vi "Main.vi"() -> ()   [LabVIEW 2009]
uses:
  C:/Code/Apps/Utilities/TunableLaserApp/Install/Samples/Labview_TLB-67xx/LabVIEW 2009/UsbDllWrap.dll
panel:
  out "Controller ID":string
  out "Serial Number:":string
  out "Model Number:":string
  out "Calibration Date:":string
  out "bScan":bool
  in  "Lambda Scan":bool
  out "bTrack":bool
  in  "Lambda Track":bool
  out "bLasPwr":bool
  in  "Laser Power":bool
  out "Error Messages":i32(listbox)
  in  "Laser Power Mode":u16(ring) caption="Laser Power" items=["Constant Current", "Constant Power"]
  in  "Stop Wavelength (nm)":dbl format="%.2g"
  in  "Start Wavelength (nm)":dbl format="%.2g"
  in  "Rev. Velocity (nm/s)":dbl format="%.2g"
  in  "Fwd. Velocity (nm/s)":dbl format="%.2g"
  in  "Desired Scans":u16
  out "Scans Completed":dbl
  in  "Piezo Voltage_Set (%)":dbl caption="Piezo Voltage (%)" format="%.2g"
  in  "Power_Set (mW)":dbl caption="Power (mW)" format="%.2g"
  in  "Current_Set (mA)":dbl caption="Current (mA)" format="%.2g"
  in  "Wavelength_Set (nm)":dbl caption="Wavelength (nm)" format="%.2g"
  out "Cavity Temp._Act (degC)":dbl caption="Cavity Temp. (degC)" format="%.2g"
  out "Diode Temp._Act (degC)":dbl caption="Diode Temp. (degC)" format="%.2g"
  out "Power_Act (mW)":dbl caption="Power (mW)" format="%.2g"
  out "Current_Act (mA)":dbl caption="Current (mA)" format="%.2g"
  out "Wavelength_Act (nm)":dbl caption="Wavelength (nm)"
  in  "Selected Controller":u16(ring) items=["6700 P1002", "TLB-6700-XP P1001"]
  # "Actual Values"
  # "Setpoint Values"
  # "Scan Settings"
  # "Mode Settings"
  # "Outputs"
  # "Laser Information"
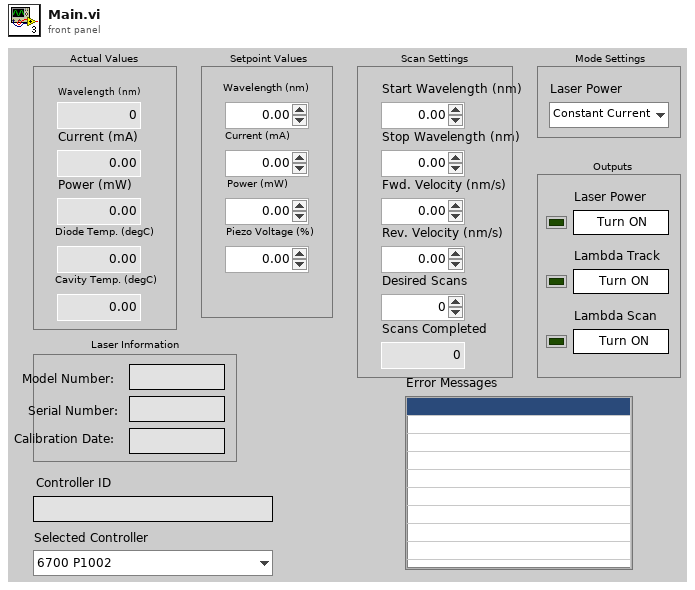
[diagram p1: front panel]
types:
  T1 = cluster{"Laser Power Mode":u16, "Start Wavelength (nm)":dbl, "Stop Wavelength (nm)":dbl, "Fwd. Velocity (nm/s)":dbl, "Rev. Velocity (nm/s)":dbl, "Desired Scans":u16, "Calibration Date:":string, "Model Number:":string, "Serial Number:":string, "Wavelength_Set (nm)":dbl, "Current_Set (mA)":dbl, "Power_Set (mW)":dbl, "Piezo Voltage_Set (%)":dbl, "Controller ID":string}
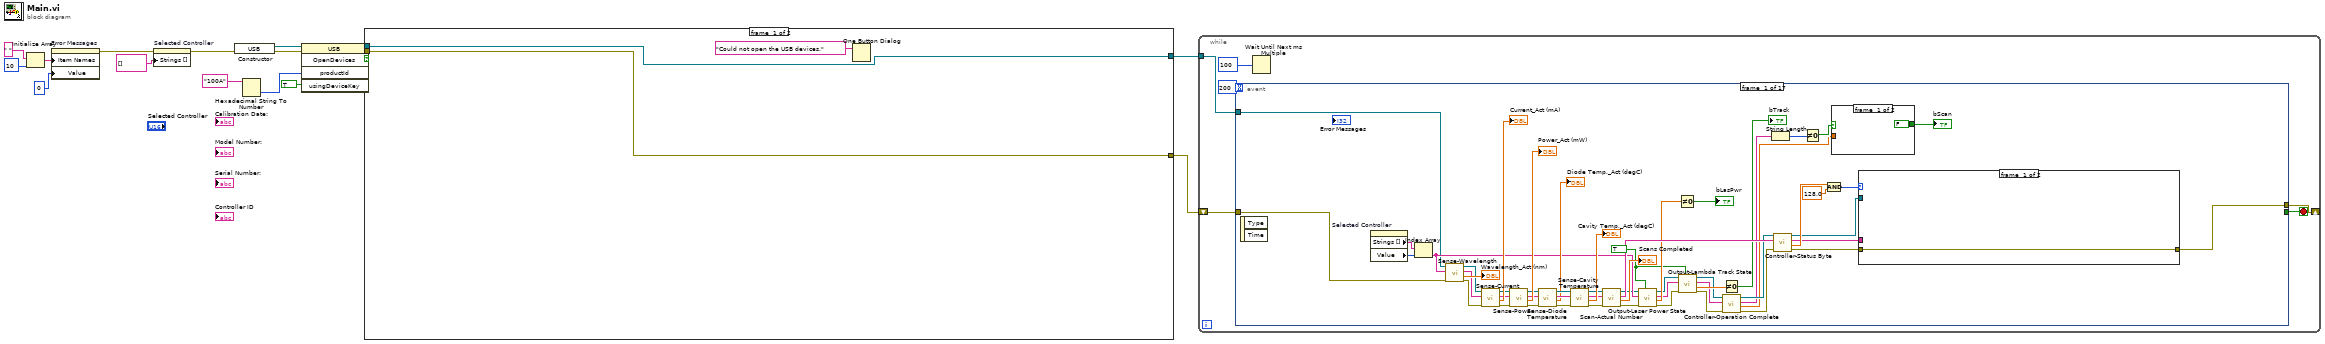
[diagram p0: block diagram]
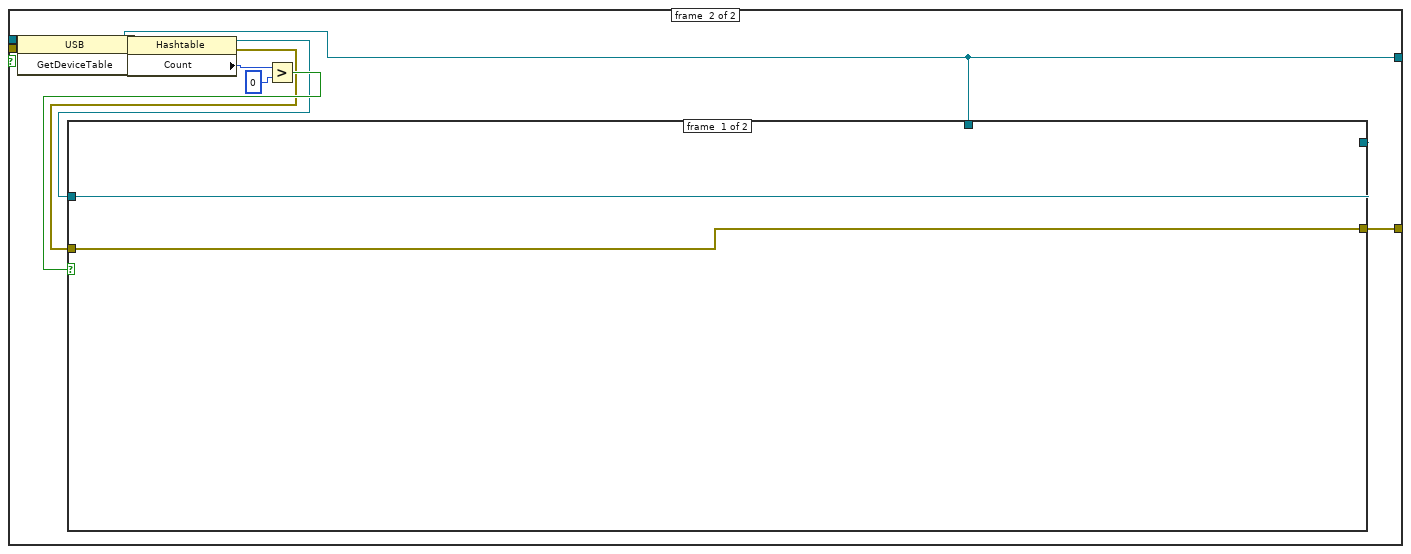
[diagram p2: hidden frame]
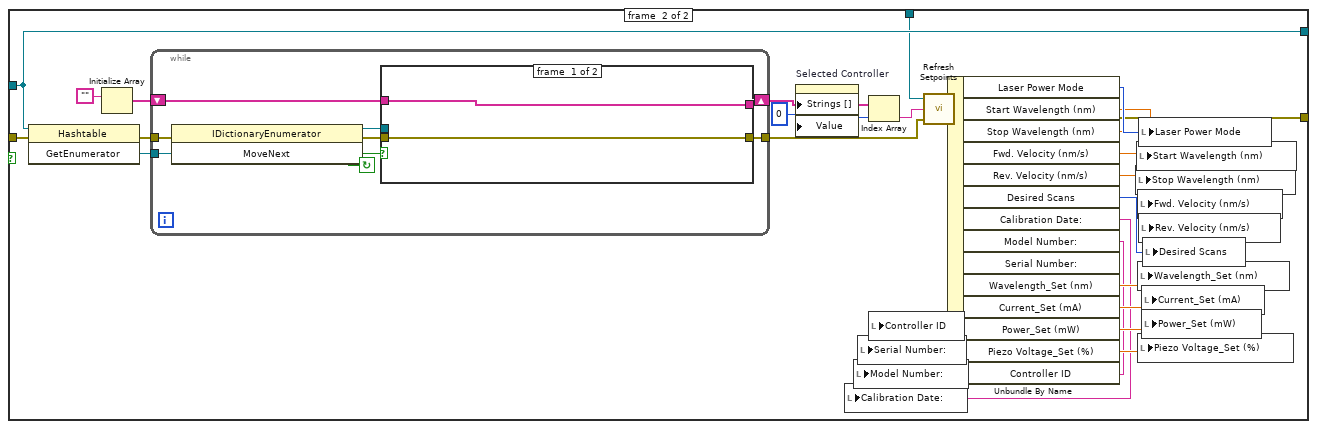
[diagram p3: hidden frame]
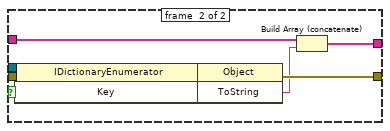
[diagram p4: hidden frame]
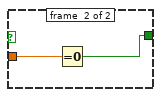
[diagram p5: hidden frame]
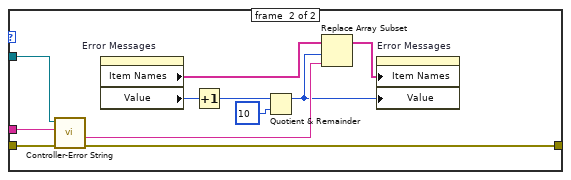
[diagram p6: hidden frame]
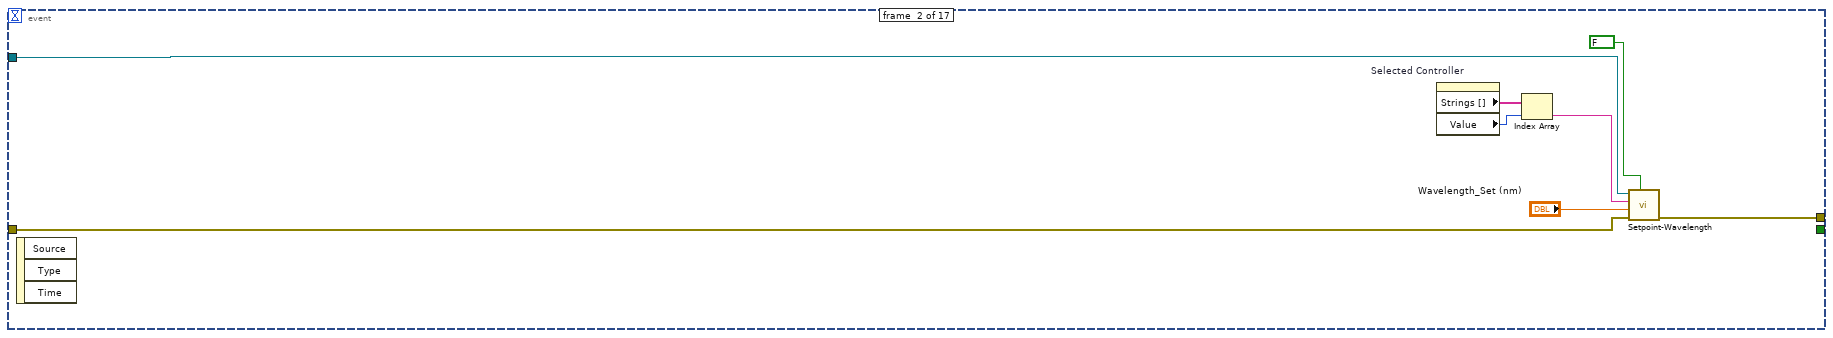
[diagram p7: hidden frame]
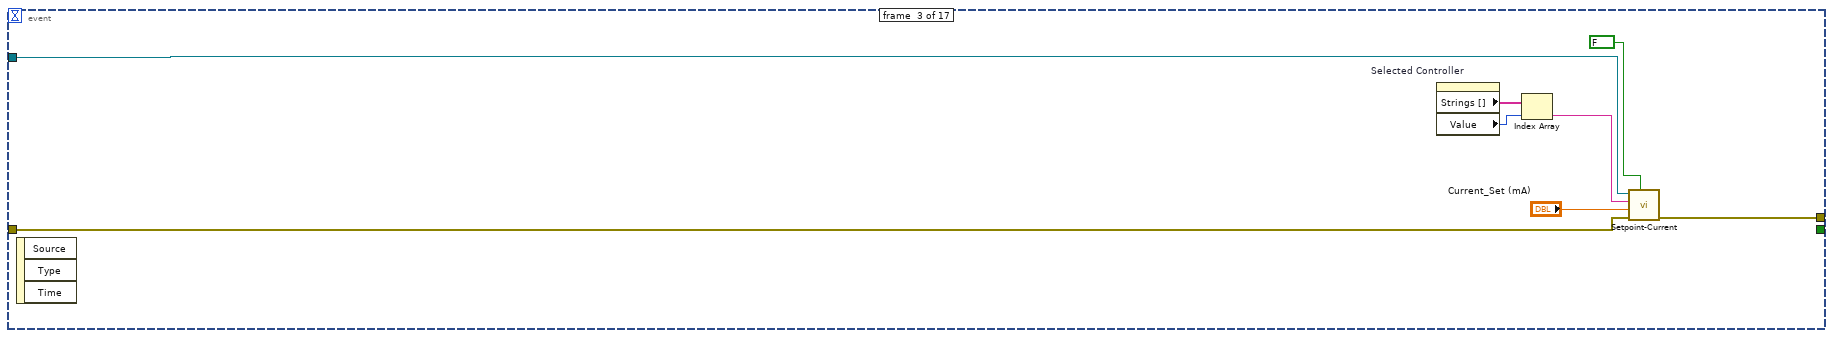
[diagram p8: hidden frame]
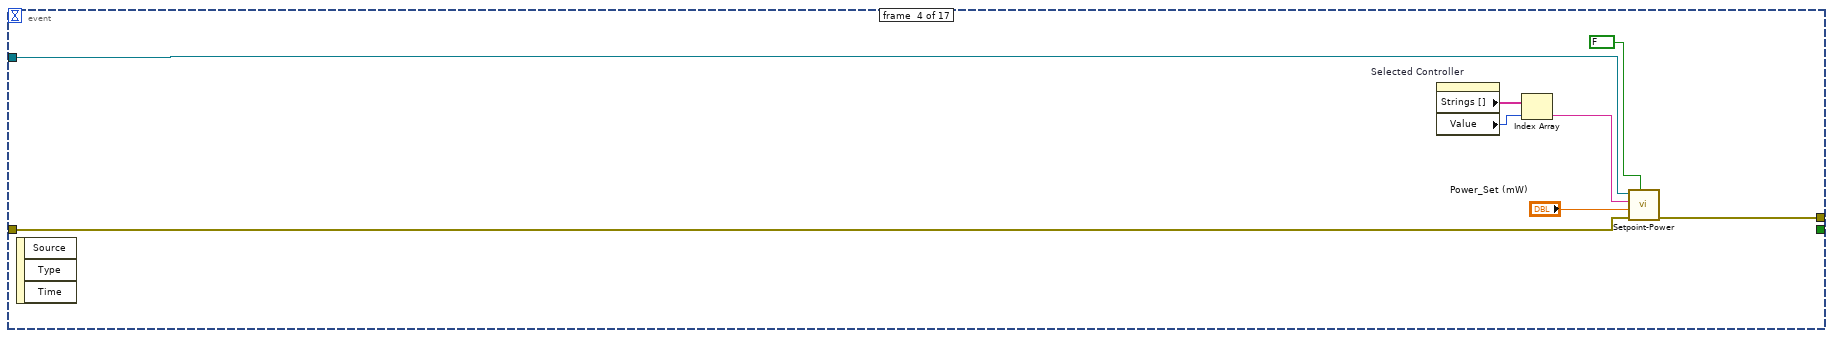
[diagram p9: hidden frame]
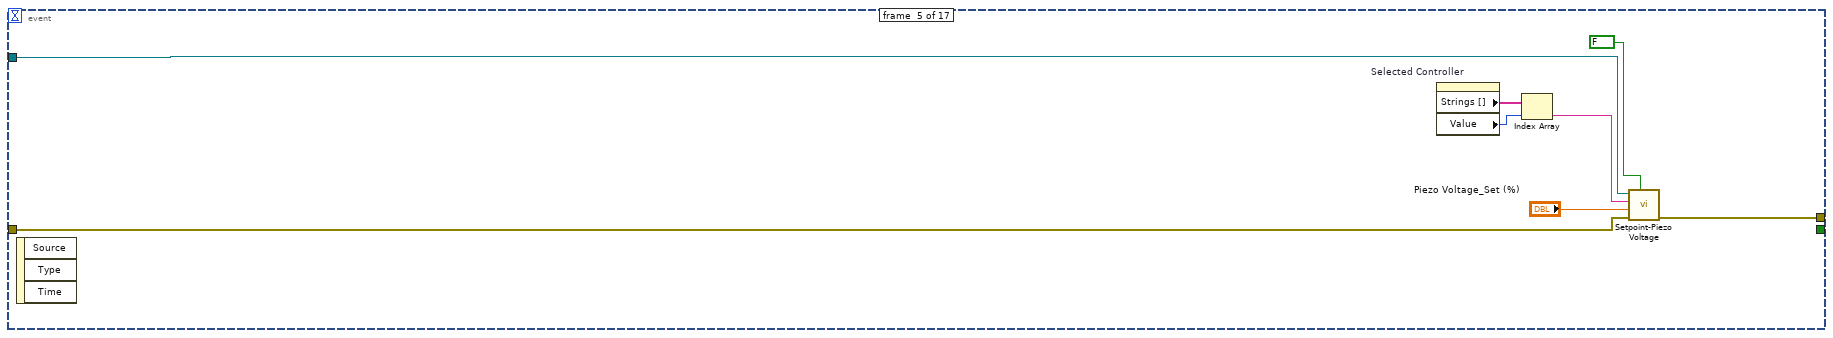
[diagram p10: hidden frame]
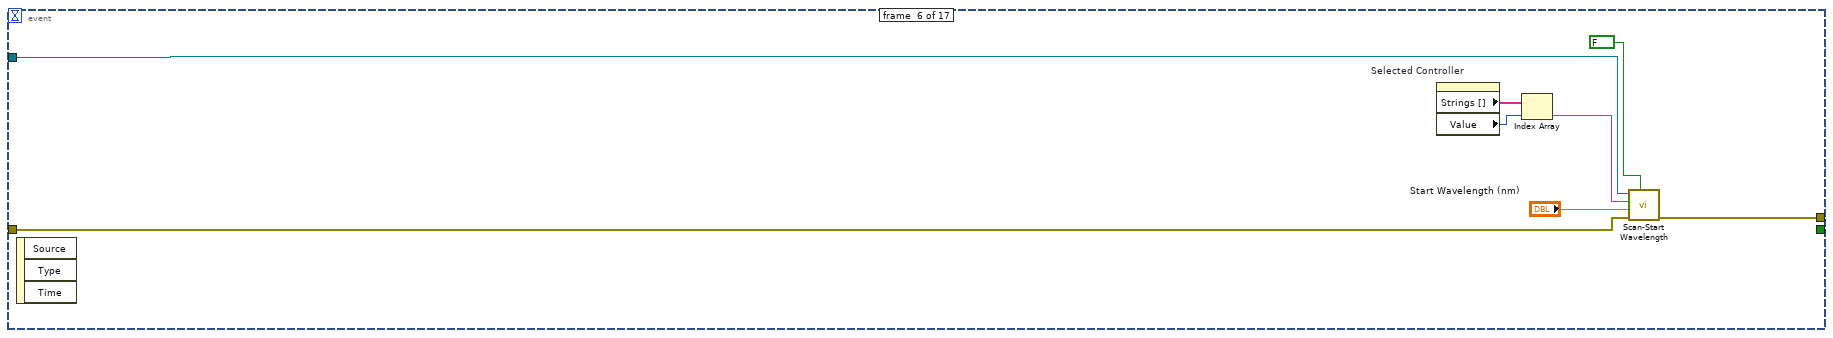
[diagram p11: hidden frame]
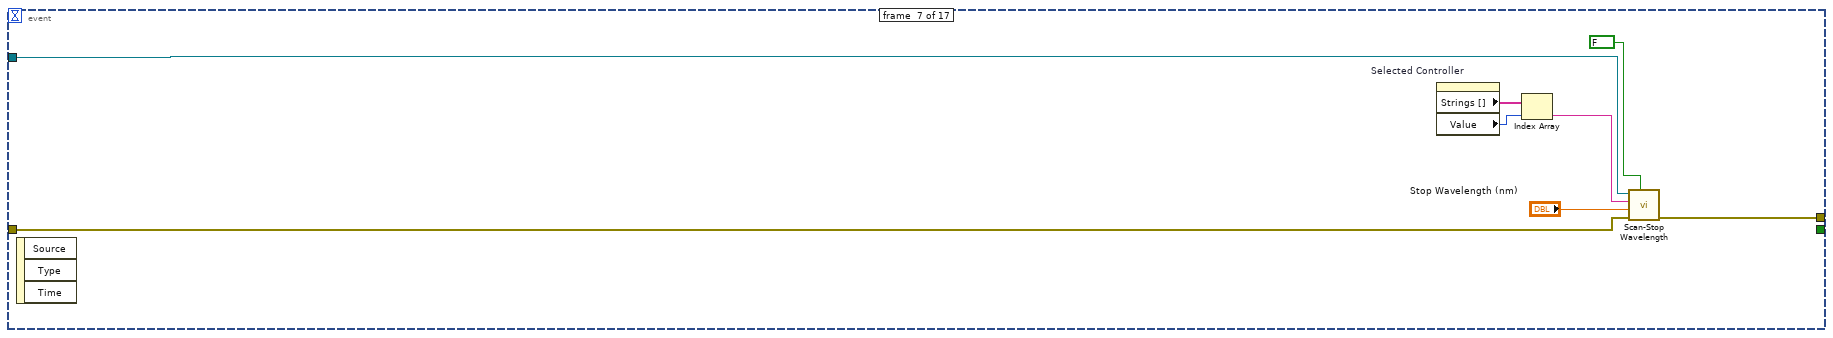
[diagram p12: hidden frame]
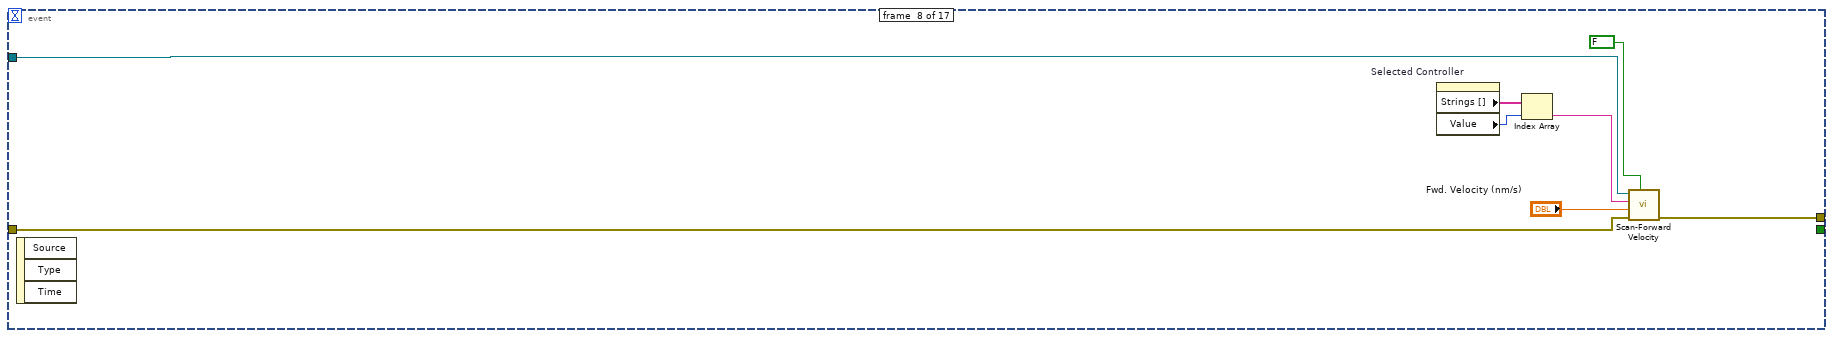
[diagram p13: hidden frame]
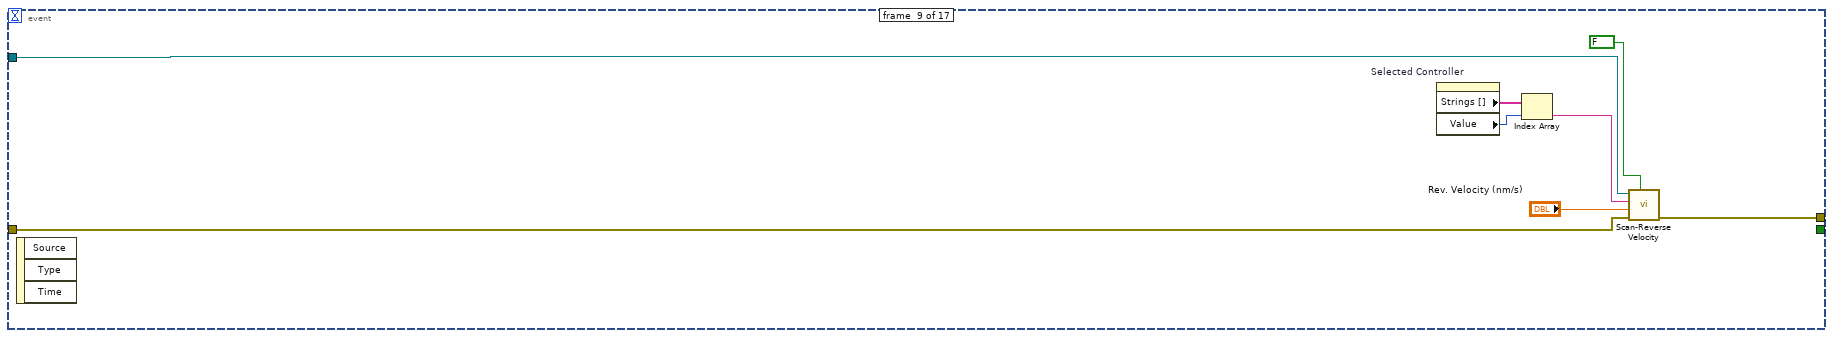
[diagram p14: hidden frame]
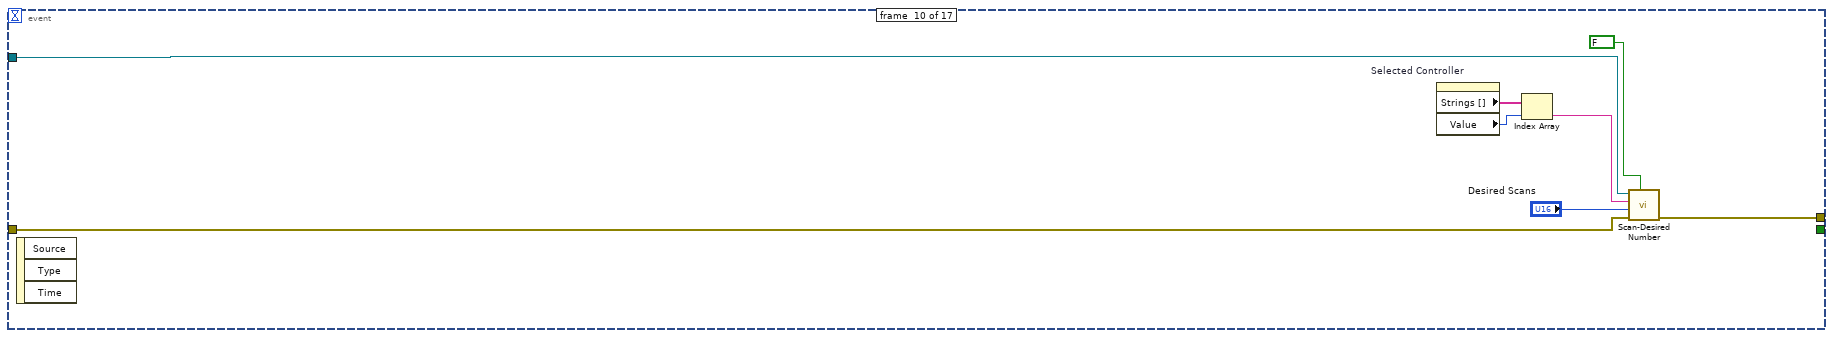
[diagram p15: hidden frame]
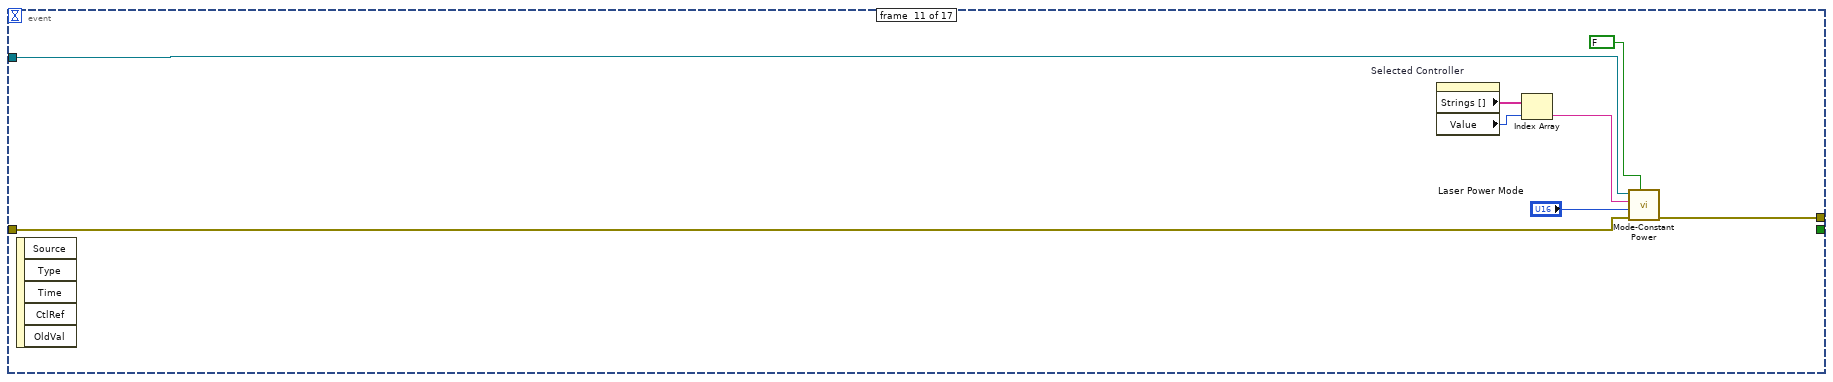
[diagram p16: hidden frame]
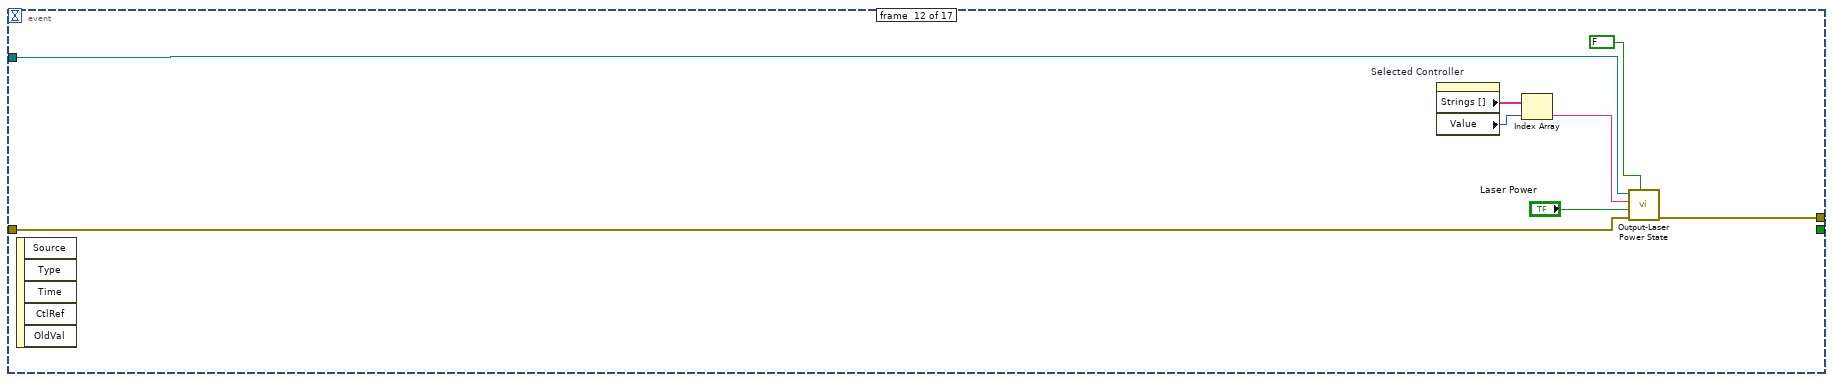
[diagram p17: hidden frame]
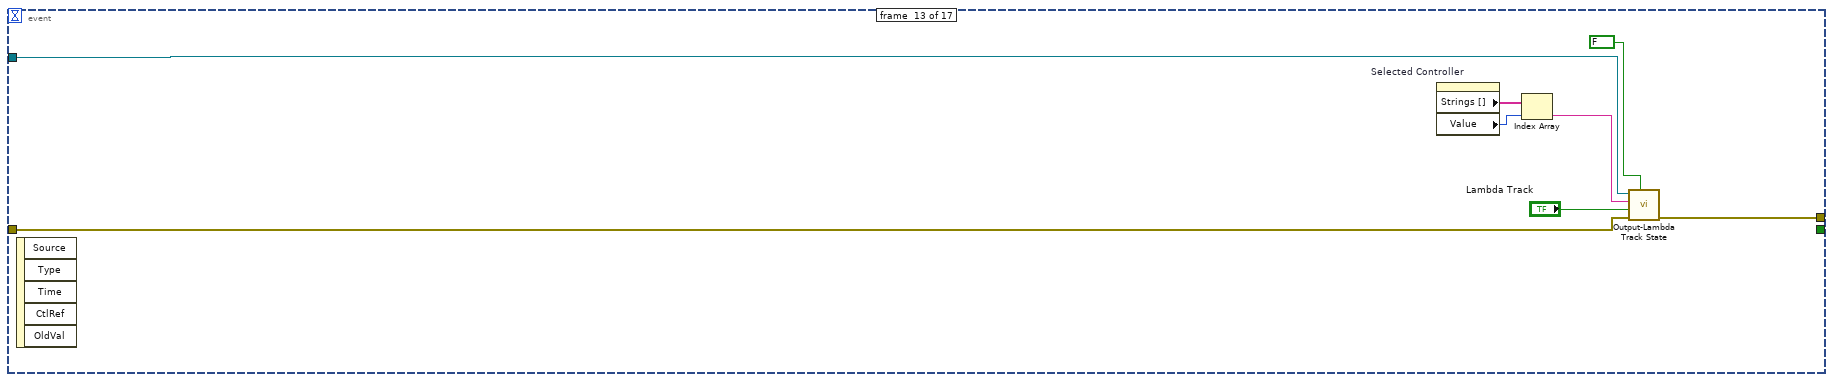
[diagram p18: hidden frame]
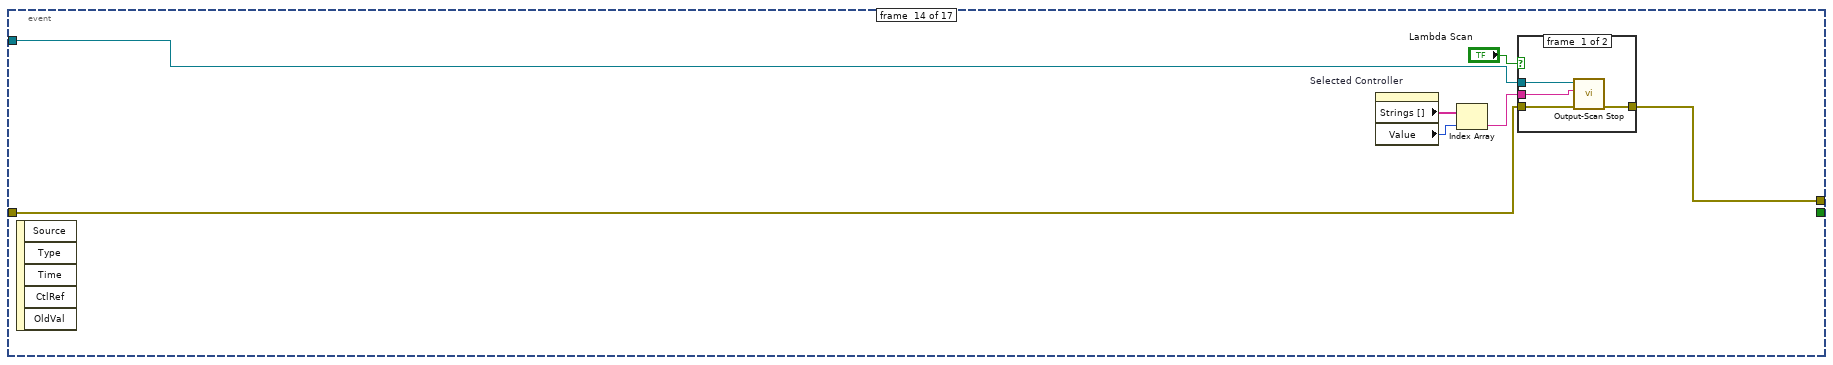
[diagram p19: hidden frame]
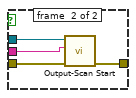
[diagram p20: hidden frame]
diagram:
  n1 = Initialize Array(" ", 10 ("dimension size")) -> (w15:string[])
  n2 = property on="Error Messages" class="LstBox (strict)"("Item Names"=w15, "Value"=0 ("Error Messages")) -> (error out=w13:errorcluster)  [unwired: 2 in, 1 out]
  n3 = property on="Selected Controller" class="Ring (strict)"(error in=w13, "Strings []"=string[] []) -> (error out=w3:errorcluster)  [unwired: 1 in, 1 out]
  n4 = constructor class="USB" ("Constructor Node")(error in=w3) -> (reference out=w9:refnum<k24>, error out=w8:errorcluster)  [unwired: 2 in, 1 out]
  n5 = Hexadecimal String To Number(string="100A") -> (number=w11:u32)  [unwired: 2 in, 1 out]
  n6 = invoke class="USB" method="OpenDevices"(reference=w9, error in=w8, "productId"=w11, "usingDeviceKey"=TRUE) -> (reference out=w4:refnum<k24>, error out=w5:errorcluster, "OpenDevices"=w6:bool)  [unwired: 1 in, 2 out]
  n7 = case shown="True" w6 {
    tunnel: w4 -> [w18 w31]
    tunnel: w5 -> [w19 w23]
    tunnel: [w19 w22] -> w1
    tunnel: [w18 w21] -> w2
    frame #0 {
      n8 = One Button Dialog(message="Could not open the USB devices.") -> ()  [unwired: 1 in, 1 out]
    }
    frame #1 {
      n9 = invoke class="USB" method="GetDeviceTable"(reference=w31, error in=w23) -> (reference out=w21:refnum<k24>, error out=w29:errorcluster, "GetDeviceTable"=w30:refnum<k24>)  [unwired: 1 in]
      n10 = property class="Hashtable"(reference=w30, error in=w29) -> (reference out=w25:refnum<k24>, error out=w24:errorcluster, "Count"=w27:i32)
      n11 = Greater?(x=w27, y=0) -> (0:w26:bool)
      n12 = case shown="True" w26 {
        tunnel: w24 -> [w33 w60]
        tunnel: w25 -> [w32 w55]
        tunnel: [w33 w34] -> w22
        tunnel: [w32 w55] -> _
        tunnel: w21 -> [_ w51]
        frame #0 {
        }
        frame #1 {
          w53 = 0
          n13 = invoke class="Hashtable" method="GetEnumerator"(reference=w55, error in=w60) -> (error out=w59:errorcluster, "GetEnumerator"=w58:refnum<k24>)  [unwired: 1 in, 1 out]
          n14 = Initialize Array("") -> (w56:string[])  [unwired: 1 in]
          n15 = while {
            tunnel: w59 -> [w68]
            tunnel: w58 -> [w67]
            tunnel: [w63] -> w35
            shift-right: [w61] -> w54
            shift-left: w56 -> [w62]
            stop <- w64 continue-if-true
            n16 = invoke class="IDictionaryEnumerator" method="MoveNext"(reference=w67, error in=w68) -> (reference out=w66:refnum<k24>, error out=w65:errorcluster, "MoveNext"=w64:bool)  [unwired: 1 in]
            n17 = case shown="True" w64 {
              tunnel: w66 -> [_ w78]
              tunnel: w65 -> [w70 w77]
              tunnel: [w70 w74] -> w63
              tunnel: w62 -> [w69 w73]
              tunnel: [w69 w71] -> w61
              frame #0 {
              }
              frame #1 {
                n18 = property class="IDictionaryEnumerator"(reference=w78, error in=w77) -> (error out=w76:errorcluster, "Key"=w75:refnum<k24>)  [unwired: 1 out]
                n19 = invoke class="Object" method="ToString"(reference=w75, error in=w76) -> (error out=w74:errorcluster, "ToString"=w72:string)  [unwired: 1 in, 1 out]
                n20 = Build Array (concatenate) "Build Array"(w73, w72) -> (w71:string[])
              }
            }
          }
          n21 = property on="Selected Controller" class="Ring (strict)"("Strings []"=w54, "Value"=w53) -> ()  [unwired: 2 in, 2 out]
          n22 = Index Array(array=w54, index=w53) -> (element=w52:string)
          n23 = call "Refresh Setpoints.vi"("error in"=w35, "DeviceKey in"=w52, "USBDLLWrap Ref In"=w51) -> ("error out"=w34:errorcluster, "Cluster"=w50:T1)
          n24 = Unbundle By Name(w50) -> ("Laser Power Mode"=w49:u16, "Start Wavelength (nm)"=w48:dbl, "Stop Wavelength (nm)"=w47:dbl, "Fwd. Velocity (nm/s)"=w46:dbl, "Rev. Velocity (nm/s)"=w45:dbl, "Desired Scans"=w44:u16, "Calibration Date:"=w39:string, "Model Number:"=w38:string, "Serial Number:"=w37:string, "Wavelength_Set (nm)"=w43:dbl, "Current_Set (mA)"=w42:dbl, "Power_Set (mW)"=w41:dbl, "Piezo Voltage_Set (%)"=w40:dbl, "Controller ID"=w36:string)
          n25 = local write "Calibration Date:"(w39) -> ()
          n26 = local write "Model Number:"(w38) -> ()
          n27 = local write "Serial Number:"(w37) -> ()
          n28 = local write "Controller ID"(w36) -> ()
          n29 = local write "Stop Wavelength (nm)"(w47) -> ()
          n30 = local write "Start Wavelength (nm)"(w48) -> ()
          n31 = local write "Fwd. Velocity (nm/s)"(w46) -> ()
          n32 = local write "Wavelength_Set (nm)"(w43) -> ()
          n33 = local write "Piezo Voltage_Set (%)"(w40) -> ()
          n34 = local write "Laser Power Mode"(w49) -> ()
          n35 = local write "Rev. Velocity (nm/s)"(w45) -> ()
          n36 = local write "Current_Set (mA)"(w42) -> ()
          n37 = local write "Power_Set (mW)"(w41) -> ()
          n38 = local write "Desired Scans"(w44) -> ()
        }
      }
    }
  }
  n39 = while {
    shift-right: [w80] -> _
    shift-left: w1 -> [w81]
    tunnel: w2 -> [w79]
    stop <- w84 stop-if-true
    n40 = event shown="[16] \"Selected Controller\": Value Change" {
      selector: _ -> [_ _ _ _ _ _ _ _ _ _ _ _ _ _ _ _ _]
      dyn-events: _ -> [_ _ _ _ _ _ _ _ _ _ _ _ _ _ _ _ _]
      timeout: 200 -> [_ _ _ _ _ _ _ _ _ _ _ _ _ _ _ _ _]
      tunnel: [_ _ _ _ _ _ _ _ _ _ _ _ _ _ TRUE TRUE _] -> w84
      tunnel: w81 -> [w119 w159 w167 w175 w183 w191 w199 w207 w215 w223 w231 w239 w247 w252 w265 w267 w270]
      tunnel: [w107 w156 w164 w172 w180 w188 w196 w204 w212 w220 w228 w236 w244 w251 w265 w267 w269] -> w80
      tunnel: w79 -> [w92 w154 w162 w170 w178 w186 w194 w202 w210 w218 w226 w234 w242 w250 _ _ w271]
      event #0 {
        w102 = TRUE ("Query?")
        n41 = event-data() -> ()  [unwired: 3 out]
        n42 = property on="Selected Controller" class="Ring (strict)"() -> ("Strings []"=w138:string[], "Value"=w137:u16)  [unwired: 2 in, 2 out]
        n43 = Index Array(array=w138, index=w137) -> (element=w106:string)
        n44 = call "Sense-Wavelength.vi"("error in"=w119, "DeviceKey in"=w106, "USBDLLWrap Ref In"=w92) -> ("error out"=w130:errorcluster, "Response"=→"Wavelength_Act (nm)":dbl, "DeviceKey out"=w134:string, "USBDLLWrap Ref Out"=w135:refnum<k24>)  [unwired: 2 out]
        n45 = call "Sense-Current.vi"("error in"=w130, "DeviceKey in"=w134, "USBDLLWrap Ref In"=w135) -> ("error out"=w129:errorcluster, "Response"=→"Current_Act (mA)":dbl, "DeviceKey out"=w131:string, "USBDLLWrap Ref Out"=w132:refnum<k24>)  [unwired: 2 out]
        n46 = call "Sense-Power.vi"("error in"=w129, "DeviceKey in"=w131, "USBDLLWrap Ref In"=w132) -> ("error out"=w127:errorcluster, "Response"=→"Power_Act (mW)":dbl, "DeviceKey out"=w126:string, "USBDLLWrap Ref Out"=w125:refnum<k24>)  [unwired: 2 out]
        n47 = call "Sense-Diode Temperature.vi"("error in"=w127, "DeviceKey in"=w126, "USBDLLWrap Ref In"=w125) -> ("error out"=w122:errorcluster, "Response"=→"Diode Temp._Act (degC)":dbl, "DeviceKey out"=w123:string, "USBDLLWrap Ref Out"=w124:refnum<k24>)  [unwired: 2 out]
        n48 = call "Sense-Cavity Temperature.vi"("error in"=w122, "DeviceKey in"=w123, "USBDLLWrap Ref In"=w124) -> ("error out"=w116:errorcluster, "Response"=→"Cavity Temp._Act (degC)":dbl, "DeviceKey out"=w117:string, "USBDLLWrap Ref Out"=w118:refnum<k24>)  [unwired: 2 out]
        n49 = call "Scan-Actual Number.vi"("error in"=w116, "DeviceKey in"=w117, "USBDLLWrap Ref In"=w118) -> ("error out"=w104:errorcluster, "Response"=→"Scans Completed":dbl, "DeviceKey out"=w114:string, "USBDLLWrap Ref Out"=w91:refnum<k24>)  [unwired: 2 out]
        n50 = call "Output-Laser Power State.vi"("Query?"=w102, "error in"=w104, "DeviceKey in"=w106, "USBDLLWrap Ref In"=w91) -> ("error out"=w98:errorcluster, "Response"=w105:dbl, "DeviceKey out"=w101:string, "USBDLLWrap Ref Out"=w103:refnum<k24>)  [unwired: 1 in]
        n51 = Not Equal To 0?(x=w105) -> (x != 0?=→"bLasPwr":bool)
        n52 = call "Output-Lambda Track State.vi"("Query?"=w102, "error in"=w98, "DeviceKey in"=w101, "USBDLLWrap Ref In"=w103) -> ("error out"=w94:errorcluster, "Response"=w100:dbl, "DeviceKey out"=w95:string, "USBDLLWrap Ref Out"=w96:refnum<k24>)  [unwired: 1 in]
        n53 = Not Equal To 0?(x=w100) -> (x != 0?=→"bTrack":bool)
        n54 = call "Controller-Operation Complete.vi"("error in"=w94, "DeviceKey in"=w95, "USBDLLWrap Ref In"=w96) -> ("error out"=w93:errorcluster, "Response"=w86:dbl, "DeviceKey out"=w89:string, "USBDLLWrap Ref Out"=w90:refnum<k24>)  [unwired: 2 out]
        n55 = String Length(string=w89) -> (length=w88:i32)
        n56 = call "Controller-Status Byte.vi"("error in"=w93, "DeviceKey in"=w114, "USBDLLWrap Ref In"=w90) -> ("error out"=w108:errorcluster, "Response"=w113:dbl, "DeviceKey out"=w109:string, "USBDLLWrap Ref Out"=w110:refnum<k24>)  [unwired: 2 out]
        n57 = Not Equal To 0?(x=w88) -> (x != 0?=w87:bool)
        n58 = Compound Arithmetic op=AND(w113, 128.0 ("value")) -> (w111:i32)
        n59 = case shown="False" w87 {
          tunnel: w86 -> [_ w141]
          tunnel: [FALSE w140] -> w85
          frame #0 {
          }
          frame #1 {
            n60 = Equal To 0?(x=w141) -> (x = 0?=w140:bool)
          }
        }
        "bScan" <- w85
        n61 = case shown="128" w111 {
          tunnel: w110 -> [_ w153]
          tunnel: w109 -> [_ w152]
          tunnel: w108 -> [w142 w151]
          tunnel: [w142 w148] -> w107
          frame #0 {
          }
          frame #1 {
            n62 = call "Controller-Error String.vi"("error in"=w151, "DeviceKey in"=w152, "USBDLLWrap Ref In"=w153) -> ("error out"=w148:errorcluster, "Response"=w147:string)  [unwired: 4 out]
            n63 = property on="Error Messages" class="LstBox (strict)"() -> ("Item Names"=w145:string[], "Value"=w144:i32)  [unwired: 2 in, 2 out]
            n64 = Increment(x=w144) -> (x+1=w150:i32)
            n65 = Quotient & Remainder(x=w150, y=10) -> (x-y*floor(x/y)=w143:i32)  [unwired: 1 out]
            n66 = Replace Array Subset(array=w145, new element=w147, index=w143) -> (w146:string[])
            n67 = property on="Error Messages" class="LstBox (strict)"("Item Names"=w146, "Value"=w143) -> ()  [unwired: 2 in, 2 out]
          }
        }
      }
      event #1 {
        n68 = event-data() -> ()  [unwired: 4 out]
        n69 = property on="Selected Controller" class="Ring (strict)"() -> ("Strings []"=w161:string[], "Value"=w160:u16)  [unwired: 2 in, 2 out]
        n70 = Index Array(array=w161, index=w160) -> (element=w157:string)
        n71 = call "Setpoint-Wavelength.vi"("Query?"=FALSE, "error in"=w159, "Wavelength (nm)"="Wavelength_Set (nm)", "DeviceKey in"=w157, "USBDLLWrap Ref In"=w154) -> ("error out"=w156:errorcluster)  [unwired: 3 out]
      }
      event #2 {
        n72 = event-data() -> ()  [unwired: 4 out]
        n73 = property on="Selected Controller" class="Ring (strict)"() -> ("Strings []"=w169:string[], "Value"=w168:u16)  [unwired: 2 in, 2 out]
        n74 = Index Array(array=w169, index=w168) -> (element=w165:string)
        n75 = call "Setpoint-Current.vi"("Query?"=FALSE, "error in"=w167, "Current (mA)"="Current_Set (mA)", "DeviceKey in"=w165, "USBDLLWrap Ref In"=w162) -> ("error out"=w164:errorcluster)  [unwired: 3 out]
      }
      event #3 {
        n76 = event-data() -> ()  [unwired: 4 out]
        n77 = property on="Selected Controller" class="Ring (strict)"() -> ("Strings []"=w177:string[], "Value"=w176:u16)  [unwired: 2 in, 2 out]
        n78 = Index Array(array=w177, index=w176) -> (element=w173:string)
        n79 = call "Setpoint-Power.vi"("Query?"=FALSE, "error in"=w175, "Power (mW)"="Power_Set (mW)", "DeviceKey in"=w173, "USBDLLWrap Ref In"=w170) -> ("error out"=w172:errorcluster)  [unwired: 3 out]
      }
      event #4 {
        n80 = event-data() -> ()  [unwired: 4 out]
        n81 = property on="Selected Controller" class="Ring (strict)"() -> ("Strings []"=w185:string[], "Value"=w184:u16)  [unwired: 2 in, 2 out]
        n82 = Index Array(array=w185, index=w184) -> (element=w181:string)
        n83 = call "Setpoint-Piezo Voltage.vi"("Query?"=FALSE, "error in"=w183, "Piezo Voltage (%)"="Piezo Voltage_Set (%)", "DeviceKey in"=w181, "USBDLLWrap Ref In"=w178) -> ("error out"=w180:errorcluster)  [unwired: 3 out]
      }
      event #5 {
        n84 = event-data() -> ()  [unwired: 4 out]
        n85 = property on="Selected Controller" class="Ring (strict)"() -> ("Strings []"=w193:string[], "Value"=w192:u16)  [unwired: 2 in, 2 out]
        n86 = Index Array(array=w193, index=w192) -> (element=w189:string)
        n87 = call "Scan-Start Wavelength.vi"("Query?"=FALSE, "error in"=w191, "Scan Start Wavelength (nm)"="Start Wavelength (nm)", "DeviceKey in"=w189, "USBDLLWrap Ref In"=w186) -> ("error out"=w188:errorcluster)  [unwired: 3 out]
      }
      event #6 {
        n88 = event-data() -> ()  [unwired: 4 out]
        n89 = property on="Selected Controller" class="Ring (strict)"() -> ("Strings []"=w201:string[], "Value"=w200:u16)  [unwired: 2 in, 2 out]
        n90 = Index Array(array=w201, index=w200) -> (element=w197:string)
        n91 = call "Scan-Stop Wavelength.vi"("Query?"=FALSE, "error in"=w199, "Scan Stop Wavelength (nm)"="Stop Wavelength (nm)", "DeviceKey in"=w197, "USBDLLWrap Ref In"=w194) -> ("error out"=w196:errorcluster)  [unwired: 3 out]
      }
      event #7 {
        n92 = event-data() -> ()  [unwired: 4 out]
        n93 = property on="Selected Controller" class="Ring (strict)"() -> ("Strings []"=w209:string[], "Value"=w208:u16)  [unwired: 2 in, 2 out]
        n94 = Index Array(array=w209, index=w208) -> (element=w205:string)
        n95 = call "Scan-Forward Velocity.vi"("Query?"=FALSE, "error in"=w207, "Scan Fwd. Vel. (nm/s)"="Fwd. Velocity (nm/s)", "DeviceKey in"=w205, "USBDLLWrap Ref In"=w202) -> ("error out"=w204:errorcluster)  [unwired: 3 out]
      }
      event #8 {
        n96 = event-data() -> ()  [unwired: 4 out]
        n97 = property on="Selected Controller" class="Ring (strict)"() -> ("Strings []"=w217:string[], "Value"=w216:u16)  [unwired: 2 in, 2 out]
        n98 = Index Array(array=w217, index=w216) -> (element=w213:string)
        n99 = call "Scan-Reverse Velocity.vi"("Query?"=FALSE, "error in"=w215, "Scan Rev. Vel. (nm/s)"="Rev. Velocity (nm/s)", "DeviceKey in"=w213, "USBDLLWrap Ref In"=w210) -> ("error out"=w212:errorcluster)  [unwired: 3 out]
      }
      event #9 {
        n100 = event-data() -> ()  [unwired: 4 out]
        n101 = property on="Selected Controller" class="Ring (strict)"() -> ("Strings []"=w225:string[], "Value"=w224:u16)  [unwired: 2 in, 2 out]
        n102 = Index Array(array=w225, index=w224) -> (element=w221:string)
        n103 = call "Scan-Desired Number.vi"("Query?"=FALSE, "error in"=w223, "Desired Number of Scans"="Desired Scans", "DeviceKey in"=w221, "USBDLLWrap Ref In"=w218) -> ("error out"=w220:errorcluster)  [unwired: 3 out]
      }
      event #10 {
        n104 = event-data() -> ()  [unwired: 6 out]
        n105 = property on="Selected Controller" class="Ring (strict)"() -> ("Strings []"=w233:string[], "Value"=w232:u16)  [unwired: 2 in, 2 out]
        n106 = Index Array(array=w233, index=w232) -> (element=w229:string)
        n107 = call "Mode-Constant Power.vi"("Query?"=FALSE, "error in"=w231, "Mode"="Laser Power Mode", "DeviceKey in"=w229, "USBDLLWrap Ref In"=w226) -> ("error out"=w228:errorcluster)  [unwired: 3 out]
      }
      event #11 {
        n108 = event-data() -> ()  [unwired: 6 out]
        n109 = property on="Selected Controller" class="Ring (strict)"() -> ("Strings []"=w241:string[], "Value"=w240:u16)  [unwired: 2 in, 2 out]
        n110 = Index Array(array=w241, index=w240) -> (element=w237:string)
        n111 = call "Output-Laser Power State.vi"("Query?"=FALSE, "error in"=w239, "Laser Power State"="Laser Power", "DeviceKey in"=w237, "USBDLLWrap Ref In"=w234) -> ("error out"=w236:errorcluster)  [unwired: 3 out]
      }
      event #12 {
        n112 = event-data() -> ()  [unwired: 6 out]
        n113 = property on="Selected Controller" class="Ring (strict)"() -> ("Strings []"=w249:string[], "Value"=w248:u16)  [unwired: 2 in, 2 out]
        n114 = Index Array(array=w249, index=w248) -> (element=w245:string)
        n115 = call "Output-Lambda Track State.vi"("Query?"=FALSE, "error in"=w247, "Lambda Track State"="Lambda Track", "DeviceKey in"=w245, "USBDLLWrap Ref In"=w242) -> ("error out"=w244:errorcluster)  [unwired: 3 out]
      }
      event #13 {
        n116 = event-data() -> ()  [unwired: 6 out]
        n117 = property on="Selected Controller" class="Ring (strict)"() -> ("Strings []"=w256:string[], "Value"=w255:u16)  [unwired: 2 in, 2 out]
        n118 = Index Array(array=w256, index=w255) -> (element=w254:string)
        n119 = case shown="True" "Lambda Scan" {
          tunnel: w250 -> [w260 w264]
          tunnel: w254 -> [w259 w263]
          tunnel: w252 -> [w258 w262]
          tunnel: [w257 w261] -> w251
          frame #0 {
            n120 = call "Output-Scan Stop.vi"("error in"=w258, "DeviceKey in"=w259, "USBDLLWrap Ref In"=w260) -> ("error out"=w257:errorcluster)  [unwired: 5 out]
          }
          frame #1 {
            n121 = call "Output-Scan Start.vi"("error in"=w262, "DeviceKey in"=w263, "USBDLLWrap Ref In"=w264) -> ("error out"=w261:errorcluster)  [unwired: 1 in, 4 out]
          }
        }
      }
      event #14 {
        n122 = event-data() -> ()  [unwired: 5 out]
        n123 = event-data() -> ()  [unwired: 1 in, 3 out]
      }
      event #15 {
        n124 = event-data() -> ()  [unwired: 4 out]
        n125 = event-data() -> ()  [unwired: 1 in, 2 out]
      }
      event #16 {
        n126 = event-data() -> ("NewVal"=w288:u16)  [unwired: 1 out]
        n127 = property on="Selected Controller" class="Ring (strict)"() -> ("Strings []"=w289:string[])  [unwired: 2 in, 2 out]
        n128 = Index Array(array=w289, index=w288) -> (element=w272:string)
        n129 = call "Refresh Setpoints.vi"("error in"=w270, "DeviceKey in"=w272, "USBDLLWrap Ref In"=w271) -> ("error out"=w269:errorcluster, "Cluster"=w287:T1)
        n130 = Unbundle By Name(w287) -> ("Laser Power Mode"=w286:u16, "Start Wavelength (nm)"=w285:dbl, "Stop Wavelength (nm)"=w284:dbl, "Fwd. Velocity (nm/s)"=w283:dbl, "Rev. Velocity (nm/s)"=w282:dbl, "Desired Scans"=w281:u16, "Calibration Date:"=w276:string, "Model Number:"=w275:string, "Serial Number:"=w274:string, "Wavelength_Set (nm)"=w280:dbl, "Current_Set (mA)"=w279:dbl, "Power_Set (mW)"=w278:dbl, "Piezo Voltage_Set (%)"=w277:dbl, "Controller ID"=w273:string)
        n131 = local write "Calibration Date:"(w276) -> ()
        n132 = local write "Model Number:"(w275) -> ()
        n133 = local write "Serial Number:"(w274) -> ()
        n134 = local write "Controller ID"(w273) -> ()
        n135 = local write "Stop Wavelength (nm)"(w284) -> ()
        n136 = local write "Start Wavelength (nm)"(w285) -> ()
        n137 = local write "Fwd. Velocity (nm/s)"(w283) -> ()
        n138 = local write "Wavelength_Set (nm)"(w280) -> ()
        n139 = local write "Piezo Voltage_Set (%)"(w277) -> ()
        n140 = local write "Laser Power Mode"(w286) -> ()
        n141 = local write "Rev. Velocity (nm/s)"(w282) -> ()
        n142 = local write "Current_Set (mA)"(w279) -> ()
        n143 = local write "Power_Set (mW)"(w278) -> ()
        n144 = local write "Desired Scans"(w281) -> ()
      }
    }
    n145 = Wait Until Next ms Multiple(millisecond multiple=u32 100) -> ()  [unwired: 1 out]
  }
